vi "Main.vi"() -> ()   [LabVIEW 2020]
uses:
  SP200-DQMH/Libraries/SP200/EC-Lab Development Package/dll_Functions.llb/OCVParameters.ctl
  Shutter-DQMH/Libraries/Shutter/Shutter State.ctl
  <vilib>/Analysis/1siggen.llb/Ramp Pattern by Delta.vi
  SMC100-DQMH/Libraries/SMC100/SMC100.lvlib
  <vilib>/Analysis/NI_AALBase.lvlib
  Shutter-DQMH/Libraries/Shutter/Shutter.lvlib
  SP200-DQMH/Libraries/SP200/SP200.lvlib
panel:
  in  "Data Interval":u32=500
  out "Current values":T1
  in  "OCV Parameters":T2={"Rest_time_T"=1.0, "Record_every_dE"=0.01, "Record_every_dT"=0.01, "E_Range"=3, "em"=1, "ce"=0, "tb"=2e-05} {"tb" min=2e-05 max=1 format="%^_3e"; "ce" items=["Standard", "CE to ground"]; "E_Range" items=["±2.5V", "±5V", "±10V", "Auto"]; "Record_every_dT" min=0 format="%.2e"; "Record_every_dE" min=0 max=100 format="%.4f"; "Rest_time_T" min=0 format="%.2f"}
  in  "Channel":u8
  out "Path_t0":path=path "D:/LabVIEW/Delay-Shutter-Sync/Time_zero.txt"
  out "Relative Delay [ps]":dbl=1.0
  out "In Backstep":bool=TRUE
  out "Backstep pos.":dbl=-2.0
  in  "Backstep Delta [ps]":dbl=-5.0
  in  "Backstep":bool=TRUE
  out "Time Remaining [min]":dbl=125.0 format="%#.1f"
  out "Estimated time total [min]":dbl=144.0 format="%#.1f"
  out "c/2 mm/ps 2":dbl=0.15
  in  "Fine Steps [ps]":dbl=0.1 format="%#_6f"
  in  "Fine End [ps]":dbl=1.0
  in  "Fine Start [ps]":dbl=-0.4999999999999953
  in  "time steps [ps]":dbl=1.0 format="%#_6f"
  out "c/2 mm/ps":dbl=0.15
  in  "End delta t [ps]":dbl=30.0 format="%#_6f"
  in  "Start delta t [ps]":dbl=-5.0
  in  "Position Time zero":dbl=14.927
  in  "CLOSED Shutter Time (s)":dbl=50.0
  in  "Fine?":bool=TRUE
  in  "Fine Steps":dbl=0.0075 format="%#_6f"
  in  "Fine End":dbl=14.62325
  in  "Fine Start":dbl=14.39825
  out "Position":dbl=14.4432
  out "Shutter State":bool
  in  "Open Shutter Panel":bool
  in  "Open Delay Stage Panel":bool
  in  "SMC100 Serial Port":u8=3
  in  "Run":bool
  out "Seconds Running":i16
  in  "OPEN Shutter Time (s)":dbl=60.0
  out "Number of Steps":i32=72
  in  "Step Size":dbl=0.075 format="%#_6f"
  in  "End Position":dbl=17.47325
  in  "Start Position":dbl=14.17325
  in  "Exit":bool=TRUE
  # "Time"
  # "Space"
  # "Current"
  # "Control"
  # "Experiment"
  # "SP-200"
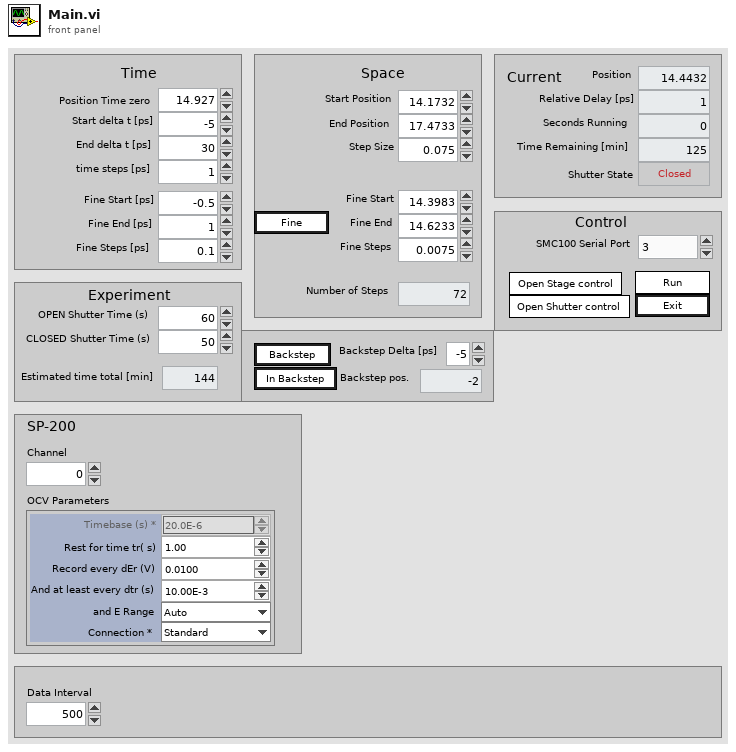
[diagram p1: front panel]
types:
  T1 = cluster{"State":i32, "MemFilled":i32, "TimeBase":sgl, " Ewe":sgl, " EweRangeMin":sgl, " EweRangeMax":sgl, "Ece":sgl, "EceRangeMin":sgl, "EceRangeMax":sgl, "Eoverflow":i32, "I":sgl, "IRange":i32, "Ioverflow":i32, "ElapsedTime":sgl, "Freq":sgl, "Rcomp":sgl, "Saturation":sgl, "OptErr":i32, "OptPos":i32}
  T2 = typedef "OCVParameters.ctl" = cluster{"Rest_time_T":sgl, "Record_every_dE":sgl, "Record_every_dT":sgl, "E_Range":u16, "em":u16, "ce":u16, "tb":sgl}
  T3 = enum32{"Invalid", "Standard", "Closed", "Hidden", "Minimized", "Maximized"}
  T4 = enum32{"invalid app kind", "Development System", "Run Time System", "Student Edition", "Embedded LabVIEW", "Evaluation", "Custom"}
  T5 = enum16{"open", "replace", "create", "open or create", "replace or create", "replace or create with confirmation"}
  T6 = typedef "Shutter State.ctl" = enum16{"None", "Open", "Closed"}
  T7 = enum8{"Enabled", "Disabled", "Disabled and Grayed Out"}
  T8 = cluster{"Core":cluster{"Current VI Reference":refnum<vi>, "Close Panel on Exit?":bool}, "Delay Positions":dbl[], "OPEN Shutter Time (s)":dbl, "Position Index":i32, "CLOSED Shutter Time (s)":dbl, "Shutter Close Time":u32, "Shutter Open Time":u32, "Save File Reference":refnum<file>}
  T9 = cluster{"Current VI Reference":refnum<vi>, "Close Panel on Exit?":bool}
  T10 = typedef "SMC100.lvlib/Get Abs Position (Reply Payload)--cluster.ctl" = cluster{"Absolute Position":dbl, "Get Abs Position_error":errorcluster}
  T11 = typedef "Shutter.lvlib/Get Shutter State (Reply Payload)--cluster.ctl" = cluster{"Shutter State":T6, "Get Shutter State_error":errorcluster}
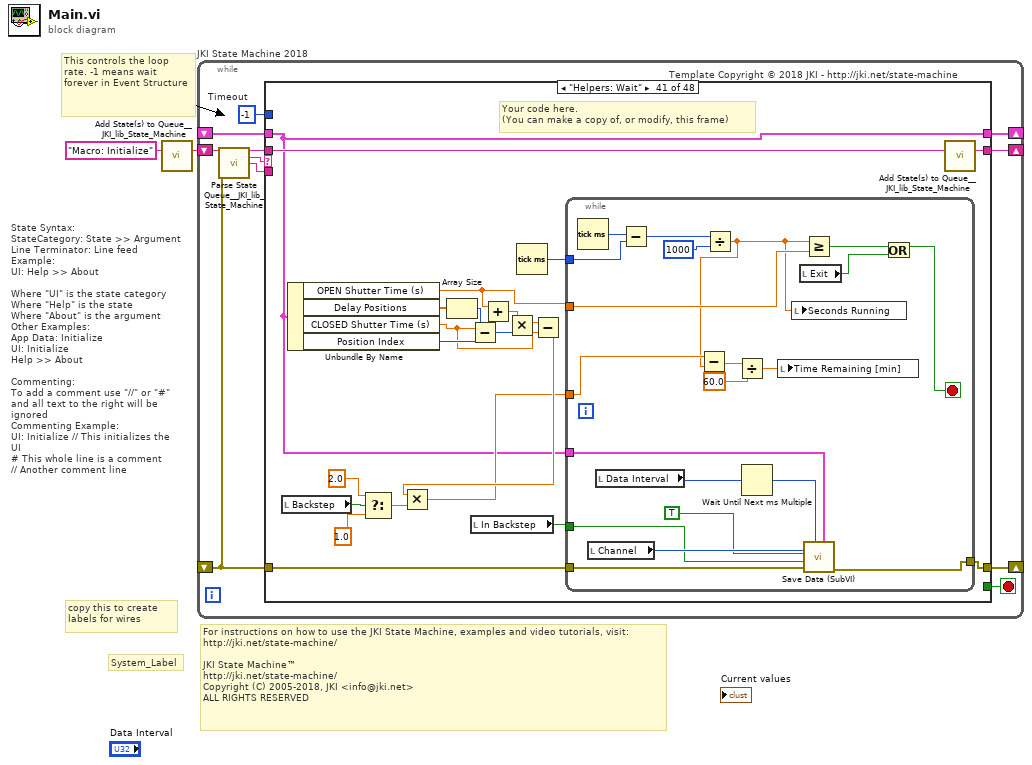
[diagram p0: block diagram]
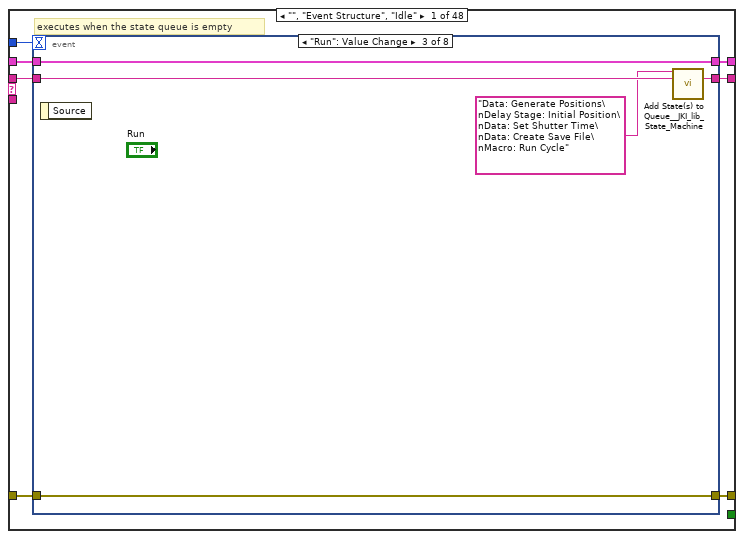
[diagram p2: hidden frame]
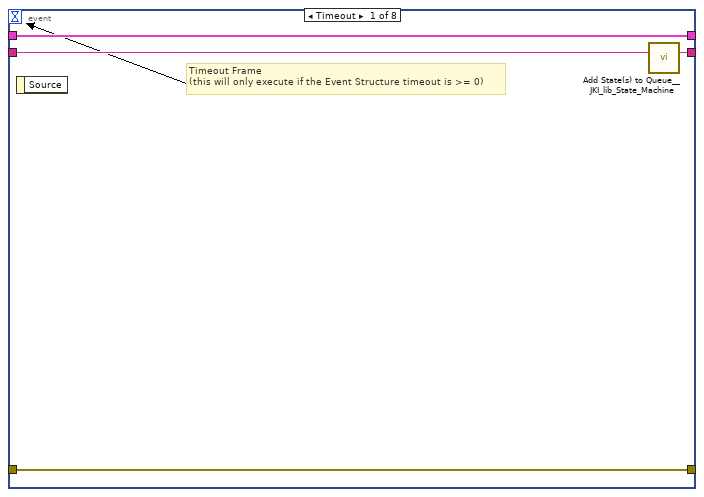
[diagram p3: hidden frame]
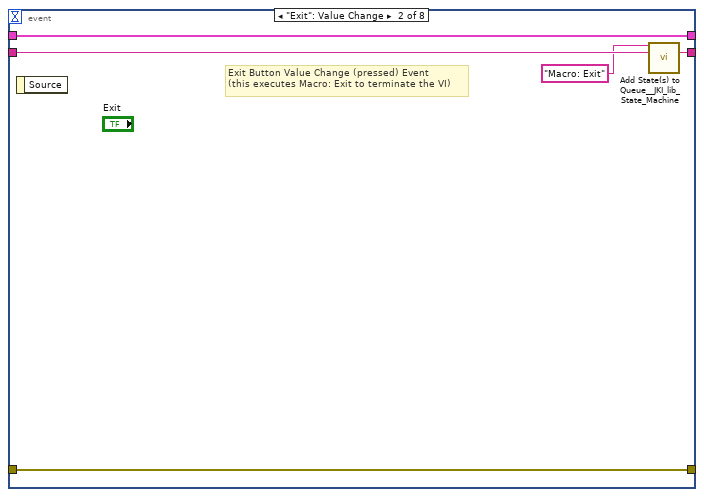
[diagram p4: hidden frame]
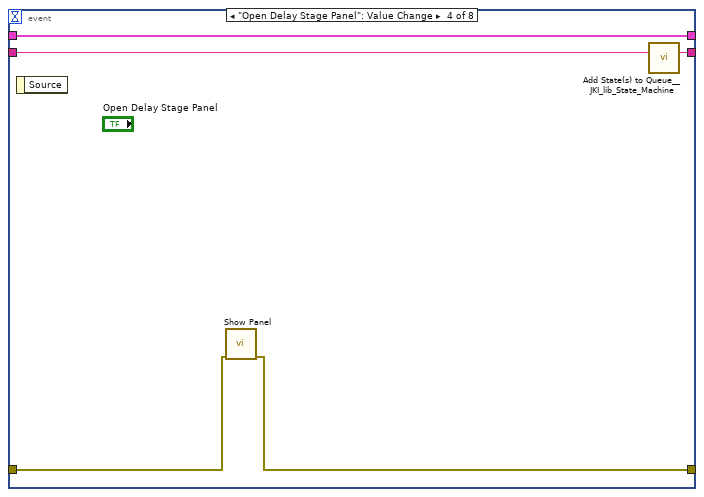
[diagram p5: hidden frame]
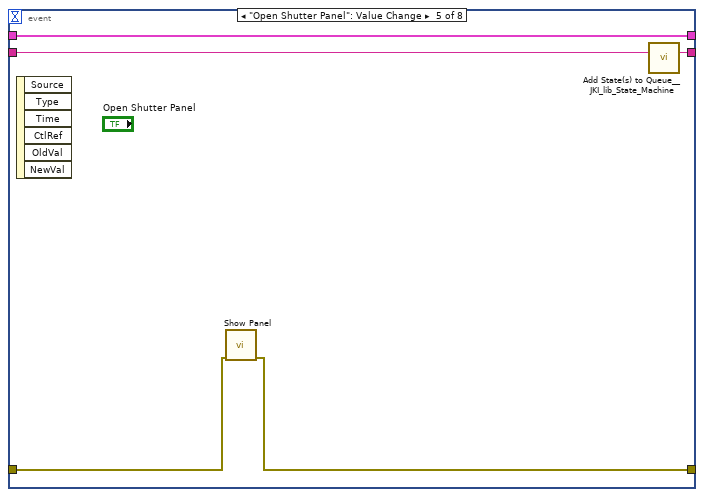
[diagram p6: hidden frame]
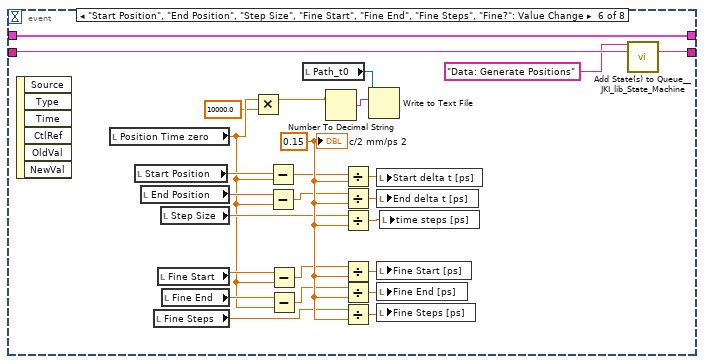
[diagram p7: hidden frame]
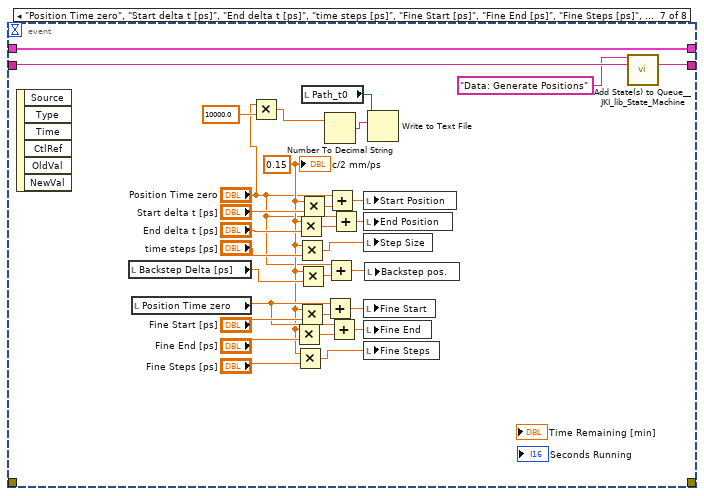
[diagram p8: hidden frame]
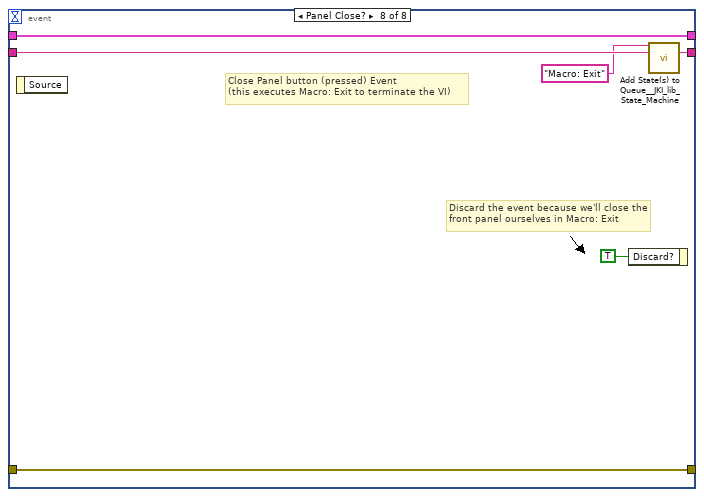
[diagram p9: hidden frame]
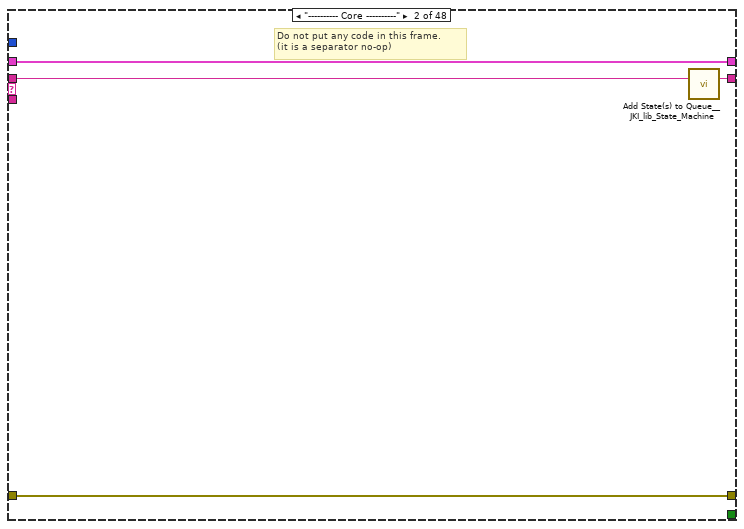
[diagram p10: hidden frame]
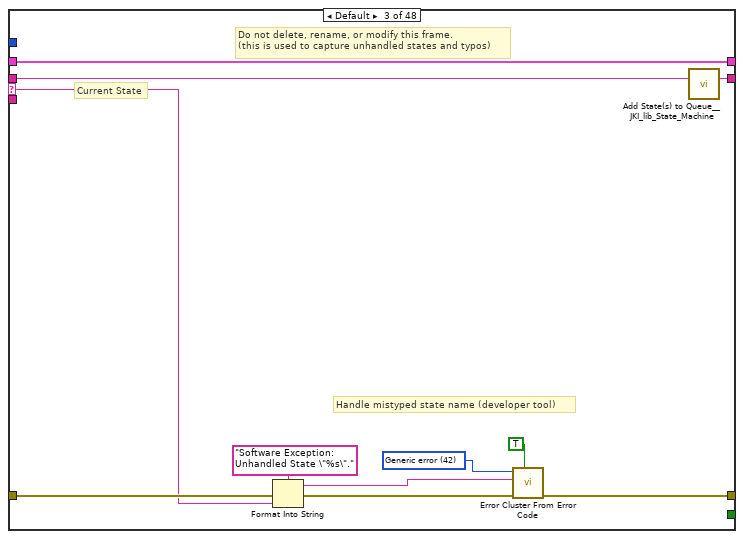
[diagram p11: hidden frame]
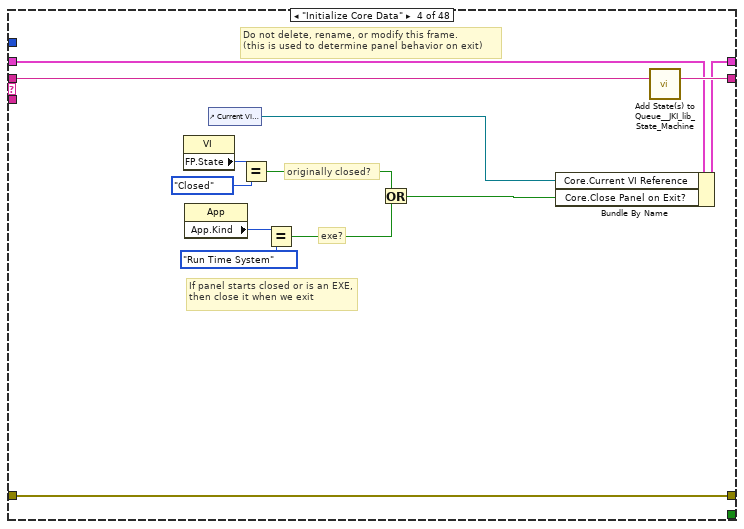
[diagram p12: hidden frame]
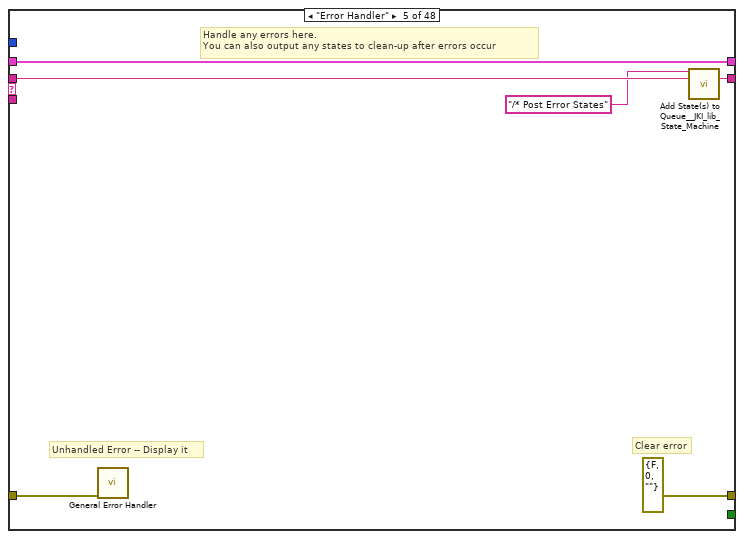
[diagram p13: hidden frame]
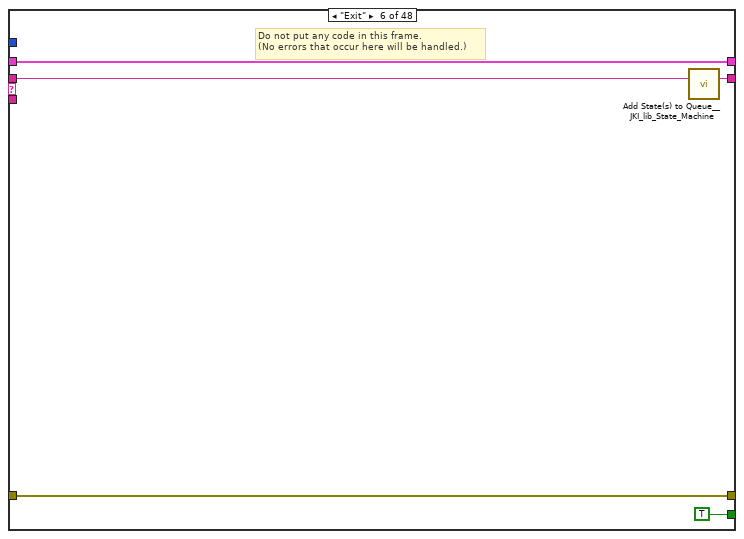
[diagram p14: hidden frame]
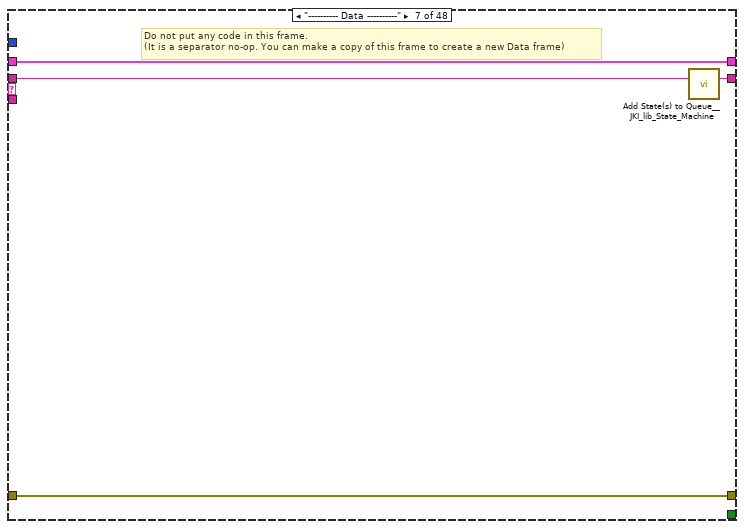
[diagram p15: hidden frame]
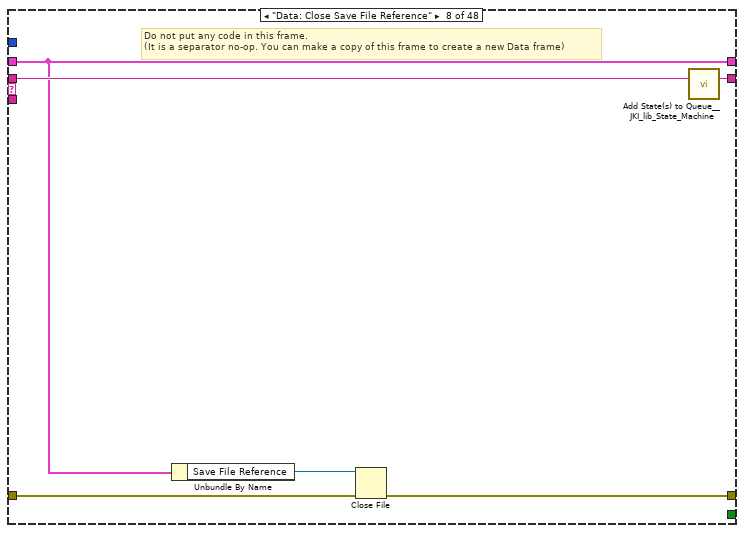
[diagram p16: hidden frame]
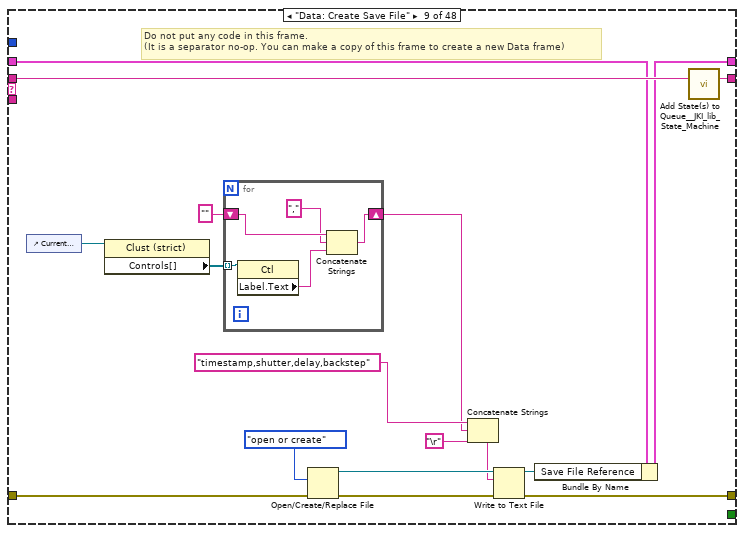
[diagram p17: hidden frame]
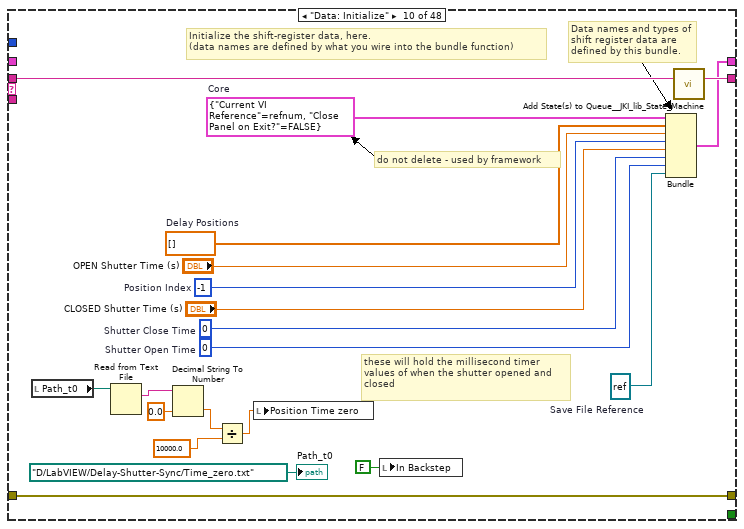
[diagram p18: hidden frame]
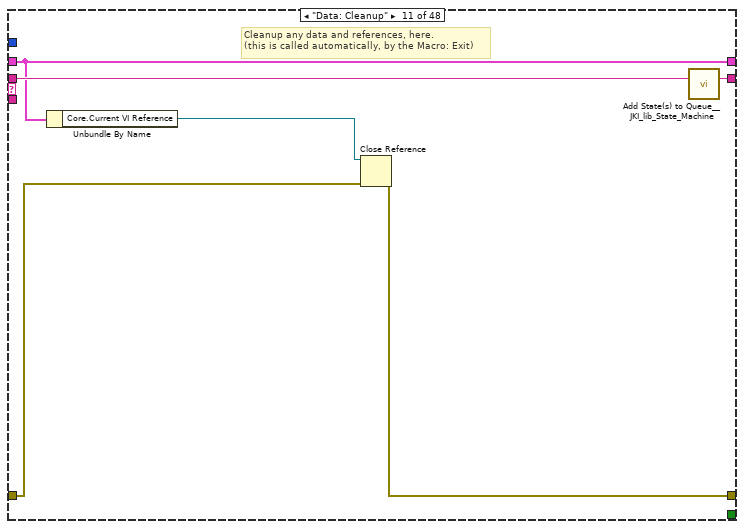
[diagram p19: hidden frame]
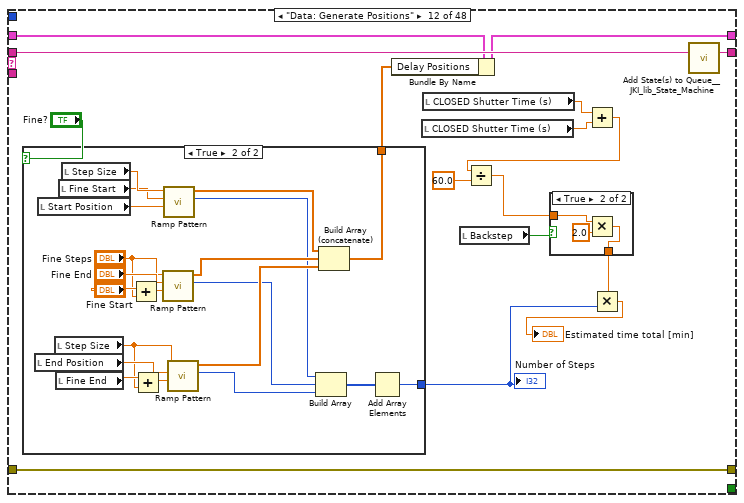
[diagram p20: hidden frame]
diagram:
  # "For instructions on how to use the JKI State Machine, examples and video tutorials, visit:\nhttp://jki.net/state-machine/\n\nJKI State Machine™\nhttp://jki.net/state-machine/\nCopyright (C) 2005-2018, JKI <info@jki.net>\nALL RIGHTS RESERVED"
  # "State Syntax:\nStateCategory: State >> Argument\nLine Terminator: Line feed\nExample:\nUI: Help >> About\n\nWhere \"UI\" is the state category\nWhere \"Help\" is the state\nWhere \"About\" is the argument\nOther Examples:\nApp Data: Initialize\nUI: Initialize\nHelp >> About\n\nCommenting:\nTo add a comment use \"//\" or \"#\" and all text to the right will be ignored\nCommenting Example:\nUI: Initialize // This initializes the UI\n# This whole line is a comment\n// Another comment line"
  # "copy this to create labels for wires"
  # "This controls the loop rate. -1 means wait forever in Event Structure"
  # "System_Label"
  n1 = call <vilib>:"Add State(s) to Queue__JKI_lib_State_Machine.vi"("State(s) in (\"\")"="Macro: Initialize") -> ("States Out"=w2:string)  [unwired: 14 in]
  n2 = while "JKI State Machine 2018" {
    shift-right: [w6] -> _
    shift-left: _ -> [w5]
    shift-right: [w9] -> _
    shift-left: _ -> [w3]
    shift-right: [w8] -> _
    shift-left: w2 -> [w10]
    stop <- w7 stop-if-true
    w4 = -1  # Timeout
    # "Template Copyright © 2018 JKI - http://jki.net/state-machine"
    n3 = call <vilib>:"Parse State Queue__JKI_lib_State_Machine.vi"("State Queue"=w10, "Error In (no error)"=w3) -> ("Remaining States"=w12:string, "Current State"=w13:string, "Arguments"=w11:string)  [unwired: 11 in]
    n4 = case shown="\"Helpers: Wait\"" w13 {
      selector: w13 -> [_ _ w111 _ _ _ _ _ _ _ _ _ _ _ _ _ _ _ _ _ _ _ _ _ _ _ _ _ _ _ _ _ _ _ _ _ _ _ _ _ _ _ _ _ _ _ _ _]
      tunnel: w12 -> [w20 w110 w115 w134 w140 w145 w149 w155 w172 w197 w203 w219 w256 w260 w264 w270 w281 w349 w355 w360 w365 w370 w375 w385 w390 w394 w400 w405 w411 w423 w435 w446 w450 w455 w460 w469 w478 w487 w491 w507 w537 w578 w603 w609 w618 w626 w631 w638]
      tunnel: w11 -> [_ _ _ _ _ _ _ _ _ _ _ _ _ _ _ w265 w275 _ _ _ _ _ _ _ _ _ _ _ _ _ _ _ _ _ _ _ _ _ _ _ _ _ _ _ _ _ _ _]
      tunnel: w5 -> [w18 w107 w113 w127 w137 w143 w146 w150 w169 _ w198 w216 w253 w257 w262 w268 w277 w348 w352 w357 w362 w367 w372 w382 w387 w391 w397 w402 w408 w419 w426 w443 w447 w452 w457 w466 w475 w485 w488 w504 w519 w561 w600 w607 w615 w623 w628 w635]
      tunnel: [w17 w108 w117 w131 errorcluster {"status"=FALSE, "code"=0, "source"=""} ("error out") w142 w147 w152 w166 w194 w199 w217 w254 w258 w261 w266 w278 w347 w353 w358 w363 w368 w373 w383 w388 w392 w396 w401 w407 w420 w432 w442 w448 w451 w456 w464 w474 w480 w489 w505 w520 w562 w601 w605 w612 w620 w627 w633] -> w9
      tunnel: w3 -> [w16 w108 w116 w131 w136 w142 w147 w153 w170 w194 w200 w217 w254 w258 w261 w267 w279 w347 w353 w358 w363 w368 w373 w383 w388 w392 w398 w403 w409 w421 w433 w444 w448 w453 w458 w467 w476 w481 w489 w505 w521 w563 w601 w606 w616 w624 w629 w636]
      tunnel: [w19 w109 w114 w133 w139 w144 w148 w154 w171 w196 w202 w218 w255 w259 w263 w269 w280 w350 w354 w359 w364 w369 w374 w384 w389 w393 w399 w404 w410 w422 w434 w445 w449 w454 w459 w468 w477 w486 w490 w506 w536 w577 w602 w608 w617 w625 w630 w637] -> w8
      tunnel: [_ _ _ _ _ TRUE _ _ _ _ _ _ _ _ _ _ _ _ _ _ _ _ _ _ _ _ _ _ _ _ _ _ _ _ _ _ _ _ _ _ _ _ _ _ _ _ _ _] -> w7
      tunnel: [w15 w107 w113 w132 w137 w143 w146 w150 w164 w195 w198 w215 w249 w257 w262 w268 w277 w348 w352 w357 w362 w367 w372 w382 w387 w391 w397 w402 w408 w417 w426 w443 w447 w452 w457 w462 w471 w485 w488 w501 w519 w561 w600 w607 w615 w623 w628 w635] -> w6
      tunnel: w4 -> [w14 _ _ _ _ _ _ _ _ _ _ _ _ _ _ _ _ _ _ _ _ _ _ _ _ _ _ _ _ _ _ _ _ _ _ _ _ _ _ _ _ _ _ _ _ _ _ _]
      frame "", "Event Structure", "Idle" {
        # "executes when the state queue is empty"
        n5 = event shown="[2] \"Run\": Value Change" {
          selector: _ -> [_ _ _ _ _ _ _ _]
          dyn-events: _ -> [_ _ _ _ _ _ _ _]
          timeout: w14 -> [_ _ _ _ _ _ _ _]
          tunnel: w20 -> [w24 w29 w34 w39 w44 w68 w98 w106]
          tunnel: [w23 w28 w33 w38 w43 w69 w99 w105] -> w19
          tunnel: w18 -> [w21 w26 w31 w37 w42 w70 w100 w103]
          tunnel: [w22 w27 w32 w36 w41 _ _ w104] -> w17
          tunnel: w16 -> [w22 w27 w32 w35 w40 _ _ w104]
          tunnel: [w21 w26 w31 w37 w42 w70 w100 w103] -> w15
          event Timeout {
            # "Timeout Frame\n(this will only execute if the Event Structure timeout is >= 0)"
            n6 = event-data() -> ()  [unwired: 1 in, 1 out]
            n7 = call <vilib>:"Add State(s) to Queue__JKI_lib_State_Machine.vi"("State(s) in (\"\")"=w24) -> ("States Out"=w23:string)  [unwired: 14 in]
          }
          event "Exit": Value Change {
            # "Exit Button Value Change (pressed) Event\n(this executes Macro: Exit to terminate the VI)"
            n8 = event-data() -> ()  [unwired: 1 in, 1 out]
            n9 = call <vilib>:"Add State(s) to Queue__JKI_lib_State_Machine.vi"("State(s) in Front (\"\")"="Macro: Exit", "State(s) in (\"\")"=w29) -> ("States Out"=w28:string)  [unwired: 13 in]
          }
          event "Run": Value Change {
            n10 = event-data() -> ()  [unwired: 1 in, 1 out]
            n11 = call <vilib>:"Add State(s) to Queue__JKI_lib_State_Machine.vi"("State(s) in Front (\"\")"="Data: Generate Positions\nDelay Stage: Initial Position\nData: Set Shutter Time\nData: Create Save File\nMacro: Run Cycle", "State(s) in (\"\")"=w34) -> ("States Out"=w33:string)  [unwired: 13 in]
          }
          event "Open Delay Stage Panel": Value Change {
            n12 = event-data() -> ()  [unwired: 1 in, 1 out]
            n13 = call "Show Panel.vi"("error in (no error)"=w35) -> ("error out"=w36:errorcluster)  [unwired: 10 in]
            n14 = call <vilib>:"Add State(s) to Queue__JKI_lib_State_Machine.vi"("State(s) in (\"\")"=w39) -> ("States Out"=w38:string)  [unwired: 14 in]
          }
          event "Open Shutter Panel": Value Change {
            n15 = event-data() -> ()  [unwired: 1 in, 6 out]
            n16 = call "Show Panel.vi"("error in (no error)"=w40) -> ("error out"=w41:errorcluster)  [unwired: 10 in]
            n17 = call <vilib>:"Add State(s) to Queue__JKI_lib_State_Machine.vi"("State(s) in (\"\")"=w44) -> ("States Out"=w43:string)  [unwired: 14 in]
          }
          event "Start Position", "End Position", "Step Size", "Fine Start", "Fine End", "Fine Steps", "Fine?": Value Change {
            w60 = 0.15 ("c mm/ps")
            n18 = event-data() -> ()  [unwired: 1 in, 6 out]
            n19 = local read "Position Time zero"() -> (w47:dbl)
            n20 = local read "Start Position"() -> (w59:dbl)
            n21 = local read "End Position"() -> (w58:dbl)
            n22 = local read "Fine Steps"() -> (w57:dbl)
            n23 = local read "Fine Start"() -> (w53:dbl)
            n24 = local read "Step Size"() -> (w56:dbl)
            n25 = local read "Fine End"() -> (w52:dbl)
            n26 = Multiply(x=w47, y=10000.0) -> (x*y=w46:dbl)
            n27 = Subtract(x=w59, y=w47) -> (x-y=w55:dbl)
            n28 = Subtract(x=w58, y=w47) -> (x-y=w54:dbl)
            n29 = Subtract(x=w53, y=w47) -> (x-y=w51:dbl)
            n30 = Subtract(x=w52, y=w47) -> (x-y=w50:dbl)
            n31 = local read "Path_t0"() -> (w48:path)
            n32 = Number To Decimal String(number=w46) -> (decimal integer string=w49:string)  [unwired: 1 in]
            n33 = Divide(x=w55, y=w60) -> (x/y=w66:dbl)
            n34 = Divide(x=w54, y=w60) -> (x/y=w64:dbl)
            n35 = Divide(x=w56, y=w60) -> (x/y=w65:dbl)
            n36 = Divide(x=w51, y=w60) -> (x/y=w61:dbl)
            n37 = Divide(x=w50, y=w60) -> (x/y=w62:dbl)
            n38 = Divide(x=w57, y=w60) -> (x/y=w63:dbl)
            n39 = Write to Text File(file (use dialog)=w48, text=w49) -> ()  [unwired: 2 in, 3 out]
            n40 = local write "Start delta t [ps]"(w66) -> ()
            n41 = local write "End delta t [ps]"(w64) -> ()
            n42 = local write "Fine Start [ps]"(w61) -> ()
            n43 = local write "Fine End [ps]"(w62) -> ()
            n44 = local write "Fine Steps [ps]"(w63) -> ()
            n45 = local write "time steps [ps]"(w65) -> ()
            n46 = call <vilib>:"Add State(s) to Queue__JKI_lib_State_Machine.vi"("State(s) in Front (\"\")"="Data: Generate Positions" ("State(s) in Front (\"\")"), "State(s) in (\"\")"=w68) -> ("States Out"=w69:string)  [unwired: 13 in]
            "c/2 mm/ps 2" <- w60
          }
          event "Position Time zero", "Start delta t [ps]", "End delta t [ps]", "time steps [ps]", "Fine Start [ps]", "Fine End [ps]", "Fine Steps [ps]", "CLOSED Shutter Time (s)", "OPEN Shutter Time (s)", "Backstep Delta [ps]": Value Change {
            w76 = 0.15 ("c mm/ps")
            n47 = event-data() -> ()  [unwired: 1 in, 6 out]
            n48 = local read "Backstep Delta [ps]"() -> (w77:dbl)
            n49 = local read "Position Time zero"() -> (w80:dbl)
            n50 = Multiply(x="Position Time zero", y=10000.0) -> (x*y=w71:dbl)
            n51 = Multiply(x=w76, y="Fine End [ps]") -> (x*y=w85:dbl)
            n52 = Multiply(x=w76, y="Fine Steps [ps]") -> (x*y=w88:dbl)
            n53 = Multiply(x=w76, y="End delta t [ps]") -> (x*y=w93:dbl)
            n54 = Multiply(x=w76, y="time steps [ps]") -> (x*y=w89:dbl)
            n55 = Multiply(x=w76, y="Fine Start [ps]") -> (x*y=w84:dbl)
            n56 = Multiply(x=w76, y=w77) -> (x*y=w78:dbl)
            n57 = Multiply(x=w76, y="Start delta t [ps]") -> (x*y=w95:dbl)
            n58 = local read "Path_t0"() -> (w74:path)
            n59 = Number To Decimal String(number=w71) -> (decimal integer string=w75:string)  [unwired: 1 in]
            n60 = Add(x=w80, y=w84) -> (x+y=w86:dbl)
            n61 = Add(x="Position Time zero", y=w78) -> (x+y=w79:dbl)
            n62 = Add(x="Position Time zero", y=w95) -> (x+y=w92:dbl)
            n63 = Add(x=w80, y=w85) -> (x+y=w87:dbl)
            n64 = Add(x="Position Time zero", y=w93) -> (x+y=w91:dbl)
            n65 = local write "Start Position"(w92) -> ()
            n66 = local write "End Position"(w91) -> ()
            n67 = local write "Step Size"(w89) -> ()
            n68 = local write "Fine Start"(w86) -> ()
            n69 = local write "Fine End"(w87) -> ()
            n70 = local write "Fine Steps"(w88) -> ()
            n71 = local write "Backstep pos."(w79) -> ()
            n72 = Write to Text File(file (use dialog)=w74, text=w75) -> ()  [unwired: 2 in, 3 out]
            n73 = call <vilib>:"Add State(s) to Queue__JKI_lib_State_Machine.vi"("State(s) in Front (\"\")"="Data: Generate Positions" ("State(s) in Front (\"\")"), "State(s) in (\"\")"=w98) -> ("States Out"=w99:string)  [unwired: 13 in]
            "c/2 mm/ps" <- w76
          }
          event Panel Close? {
            # "Discard the event because we'll close the front panel ourselves in Macro: Exit"
            # "Close Panel button (pressed) Event\n(this executes Macro: Exit to terminate the VI)"
            n74 = event-data() -> ()  [unwired: 1 in, 1 out]
            n75 = event-data("Discard?"=TRUE) -> ()  [unwired: 1 in, 1 out]
            n76 = call <vilib>:"Add State(s) to Queue__JKI_lib_State_Machine.vi"("State(s) in Front (\"\")"="Macro: Exit", "State(s) in (\"\")"=w106) -> ("States Out"=w105:string)  [unwired: 13 in]
          }
        }
      }
      frame "---------- Core ----------" {
        # "Do not put any code in this frame.\n(it is a separator no-op)"
        n77 = call <vilib>:"Add State(s) to Queue__JKI_lib_State_Machine.vi"("State(s) in (\"\")"=w110) -> ("States Out"=w109:string)  [unwired: 14 in]
      }
      frame Default {
        w120 = 42 items=["No error", "Argument error", "Memory is full", "Out of zone", "End of file", "File already open", "Generic file I/O error", "File not found", "File permission error", "Disk is full", "Duplicate path", "Too many files open", "System feature not enabled", "Resource file not found", "Cannot add resource", "Resource not found", "Image not found", "Image memory error", "Pen does not exist", "Config type invalid", "Config token not found", "Config parse error", "Config memory error", "Bad external code format", "Bad external code offset", "External code not present", "Null window", "Destroy window error", "Null menu", "Print aborted", "Bad print record", "Print driver error", "Windows error during printing", "Memory error during printing", "Print dialog error", "Generic print error", "Invalid device refnum", "Device not found", "Device parameter error", "Device unit error", "Cannot open device", "Device call aborted", "Generic error", "Cancelled by user", "Object ID too low", "Object ID too high", "Object not in heap", "Unknown heap", "Unknown object (invalid DefProc)", "Unknown object (DefProc not in table)", "Message out of range", "Invalid (null) method", "Unknown message", "Manager call not supported", "Bad address", "Network operation in progress", "Network operation timed out", "Connection is busy", "Network attribute not supported", "Network error", "Address in use", "System out of memory", "Connection aborted", "Connection refused", "Not connected", "Already connected", "Connection closed", "Initialization error (interapplication manager)", "Bad occurrence", "Wait on unbound occurrence handler", "Occurrence queue overflow", "Datalog type conflict", "Unused", "Unrecognized type (interapplication manager)", "Memory corrupt", "Failed to make temporary DLL", "Old CIN version", "Drag socket not found", "Failed to load drop-object", "Failed to register OLE object", "Failed to release OLE object", "Format specifier type mismatch", "Unknown format specifier", "Too few format specifiers", "Too many format specifiers", "Scan failed", "Newer CIN version", "Error converting to variant", "Runtime menu error", "Password tampered", "Variant attribute not found", "Incompatible variant data type", "Event data is not available", "Event Store is not present", "Occurrence is not found", "Event Queue is not created", "Event info is not available", "Refnum passed is NULL", "Error retrieving Class GUID", "Error retrieving CoClass GUID", "Error retrieving TypeLib GUID.", "Bad built application magic bytes.", "Specific driver is different from the specific driver associated with the Logical Name.", "There is no session opened to the class driver.", "Max Error", "MAX - Error with config objects", "MAX - Error loading configuration", "MAX - Group not supported"]
        # "Current State"
        # "Do not delete, rename, or modify this frame.\n(this is used to capture unhandled states and typos)"
        # "Handle mistyped state name (developer tool)"
        n78 = Format Into String(format string="Software Exception: Unhandled State \"%s\"." ("message"), error in=w116, w111) -> (resulting string=w119:string, error out=w118:errorcluster)  [unwired: 1 in]
        n79 = call <vilib>:"Error Cluster From Error Code.vi"("show call chain? (False)"=TRUE, "error in (no error)"=w118, "error message (\"\")"=w119, "error code (0)"=w120) -> ("error out"=w117:errorcluster)  [unwired: 5 in]
        n80 = call <vilib>:"Add State(s) to Queue__JKI_lib_State_Machine.vi"("State(s) in (\"\")"=w115) -> ("States Out"=w114:string)  [unwired: 14 in]
      }
      frame "Initialize Core Data" {
        # "Do not delete, rename, or modify this frame.\n(this is used to determine panel behavior on exit)"
        # "originally closed?"
        # "exe?"
        # "If panel starts closed or is an EXE, then close it when we exit"
        n81 = property class="VI"() -> ("FP.State"=w124:T3)  [unwired: 2 in, 2 out]
        n82 = property class="App"() -> ("App.Kind"=w130:T4)  [unwired: 2 in, 2 out]
        n83 = control-ref of="Current VI Reference"() -> (w125:refnum<vi>)
        n84 = Equal?(x=w124, y=T3."Closed" ("Front Panel Window:State")) -> (x = y?=w122:bool)
        n85 = Equal?(x=w130, y=T4."Run Time System" ("Application:Kind")) -> (x = y?=w128:bool)
        n86 = Or(x=w122, y=w128) -> (x .or. y?=w126:bool)
        n87 = Bundle By Name(cluster=w127, "Core.Current VI Reference"=w125, "Core.Close Panel on Exit?"=w126) -> (w132:T8)
        n88 = call <vilib>:"Add State(s) to Queue__JKI_lib_State_Machine.vi"("State(s) in (\"\")"=w134) -> ("States Out"=w133:string)  [unwired: 14 in]
      }
      frame "Error Handler" {
        # "Unhandled Error -- Display it"
        # "Handle any errors here.\nYou can also output any states to clean-up after errors occur"
        # "Clear error"
        n89 = call <vilib>:"General Error Handler.vi"("error in (no error)"=w136) -> ()  [unwired: 10 in, 5 out]
        n90 = call <vilib>:"Add State(s) to Queue__JKI_lib_State_Machine.vi"("State(s) in Front (\"\")"="/* Post Error States", "State(s) in (\"\")"=w140) -> ("States Out"=w139:string)  [unwired: 13 in]
      }
      frame "Exit" {
        # "Do not put any code in this frame.\n(No errors that occur here will be handled.)"
        n91 = call <vilib>:"Add State(s) to Queue__JKI_lib_State_Machine.vi"("State(s) in (\"\")"=w145) -> ("States Out"=w144:string)  [unwired: 14 in]
      }
      frame "---------- Data ----------" {
        # "Do not put any code in this frame.\n(It is a separator no-op. You can make a copy of this frame to create a new Data frame)"
        n92 = call <vilib>:"Add State(s) to Queue__JKI_lib_State_Machine.vi"("State(s) in (\"\")"=w149) -> ("States Out"=w148:string)  [unwired: 14 in]
      }
      frame "Data: Close Save File Reference" {
        # "Do not put any code in this frame.\n(It is a separator no-op. You can make a copy of this frame to create a new Data frame)"
        n93 = Unbundle By Name(w150) -> ("Save File Reference"=w151:refnum<file>)
        n94 = Close File(refnum=w151, error in=w153) -> (error out=w152:errorcluster)  [unwired: 1 out]
        n95 = call <vilib>:"Add State(s) to Queue__JKI_lib_State_Machine.vi"("State(s) in (\"\")"=w155) -> ("States Out"=w154:string)  [unwired: 14 in]
      }
      frame "Data: Create Save File" {
        # "Do not put any code in this frame.\n(It is a separator no-op. You can make a copy of this frame to create a new Data frame)"
        n96 = control-ref of="Current values"() -> (w162:refnum<vi>)
        n97 = property class="Clust (strict)"(reference=w162) -> ("Controls[]"=w161:refnum<vi>[])  [unwired: 1 in, 2 out]
        n98 = for {
          tunnel: w161 -> [w177] mode=indexing
          shift-right: [w176] -> w158
          shift-left: "" -> [w175]
          n99 = property class="Ctl"(reference=w177) -> ("Label.Text"=w173:string)  [unwired: 1 in, 2 out]
          n100 = Concatenate Strings(w175, "," ("string"), w173) -> (w176:string)
        }
        n101 = Open/Create/Replace File(error in=w170, operation (0:open)=T5."open or create") -> (refnum out=w165:refnum<file>, error out=w168:errorcluster)  [unwired: 4 in, 1 out]
        n102 = Concatenate Strings("timestamp,shutter,delay,backstep" ("text"), w158, "\r") -> (w156:string)
        n103 = Write to Text File(file (use dialog)=w165, text=w156, error in=w168) -> (refnum out=w163:refnum<file>, error out=w166:errorcluster)  [unwired: 1 in, 1 out]
        n104 = Bundle By Name(cluster=w169, "Save File Reference"=w163) -> (w164:T8)
        n105 = call <vilib>:"Add State(s) to Queue__JKI_lib_State_Machine.vi"("State(s) in (\"\")"=w172) -> ("States Out"=w171:string)  [unwired: 14 in]
      }
      frame "Data: Initialize" {
        w178 = refnum<file> refnum  # Save File Reference
        w179 = u32 0  # Shutter Open Time
        w180 = u32 0  # Shutter Close Time
        w191 = -1  # Position Index
        w192 = dbl[] []  # Delay Positions
        w193 = T9 {"Current VI Reference"=refnum, "Close Panel on Exit?"=FALSE}  # Core
        # "these will hold the millisecond timer\nvalues of when the shutter opened and\nclosed"
        # "do not delete - used by framework"
        # "Data names and types of shift register data are defined by this bundle."
        # "Initialize the shift-register data, here.\n(data names are defined by what you wire into the bundle function)"
        n106 = local read "Path_t0"() -> (w186:path)
        n107 = Read from Text File(file (use dialog)=w186) -> (text=w185:string)  [unwired: 3 in, 3 out]
        n108 = Decimal String To Number(string=w185, default (0L)=0.0 ("default (0 I32)")) -> (number=w183:dbl)  [unwired: 1 in, 1 out]
        n109 = Divide(x=w183, y=10000.0 ("x/y")) -> (x/y=w182:dbl)
        n110 = local write "Position Time zero"(w182) -> ()
        n111 = local write "In Backstep"(FALSE ("In Backstep")) -> ()
        n112 = Bundle("Core"=w193, "Delay Positions"=w192, "OPEN Shutter Time (s)"="OPEN Shutter Time (s)", "Position Index"=w191, "CLOSED Shutter Time (s)"="CLOSED Shutter Time (s)", "Shutter Close Time"=w180, "Shutter Open Time"=w179, "Save File Reference"=w178) -> (w195:T8)  [unwired: 1 in]
        n113 = call <vilib>:"Add State(s) to Queue__JKI_lib_State_Machine.vi"("State(s) in (\"\")"=w197) -> ("States Out"=w196:string)  [unwired: 14 in]
        "Path_t0" <- path "D:/LabVIEW/Delay-Shutter-Sync/Time_zero.txt" ("file (use dialog)")
      }
      frame "Data: Cleanup" {
        # "Cleanup any data and references, here.\n(this is called automatically, by the Macro: Exit)"
        n114 = Unbundle By Name(w198) -> ("Core.Current VI Reference"=w201:refnum<vi>)
        n115 = Close Reference(reference=w201, error in (no error)=w200) -> (error out=w199:errorcluster)
        n116 = call <vilib>:"Add State(s) to Queue__JKI_lib_State_Machine.vi"("State(s) in (\"\")"=w203) -> ("States Out"=w202:string)  [unwired: 14 in]
      }
      frame "Data: Generate Positions" {
        n117 = case shown="True" "Fine?" {
          tunnel: [w225 w230] -> w208
          tunnel: [w224 w229] -> w213
          frame False {
            n118 = local read "Start Position"() -> (w226:dbl)
            n119 = call-poly <vilib>:"Ramp Pattern.vi"("start"=w226, "end"="End Position", "delta"="Step Size") -> ("samples"=w225:i32, "Ramp Pattern"=w224:dbl[])  [unwired: 6 in, 1 out]
          }
          frame True {
            n120 = local read "End Position"() -> (w241:dbl)
            n121 = local read "Start Position"() -> (w246:dbl)
            n122 = local read "Step Size"() -> (w238:dbl)
            n123 = local read "Fine End"() -> (w240:dbl)
            n124 = local read "Fine Start"() -> (w244:dbl)
            n125 = local read "Step Size"() -> (w245:dbl)
            n126 = Add(x="Fine Start", y="Fine Steps") -> (x+y=w243:dbl)
            n127 = Add(x=w240, y=w238) -> (x+y=w239:dbl)
            n128 = call-poly <vilib>:"Ramp Pattern.vi"("start"=w243, "end"="Fine End", "delta"="Fine Steps") -> ("samples"=w233:i32, "Ramp Pattern"=w236:dbl[])  [unwired: 6 in, 1 out]
            n129 = call-poly <vilib>:"Ramp Pattern.vi"("start"=w246, "end"=w244, "delta"=w245) -> ("samples"=w232:i32, "Ramp Pattern"=w237:dbl[])  [unwired: 6 in, 1 out]
            n130 = call-poly <vilib>:"Ramp Pattern.vi"("start"=w239, "end"=w241, "delta"=w238) -> ("samples"=w234:i32, "Ramp Pattern"=w235:dbl[])  [unwired: 6 in, 1 out]
            n131 = Build Array(w232, w233, w234) -> (w231:i32[])
            n132 = Build Array (concatenate)(w237, w236, w235) -> (w229:dbl[])
            n133 = Add Array Elements(numeric array=w231) -> (sum=w230:i32)
          }
        }
        "Number of Steps" <- w208
        n134 = Bundle By Name(cluster=w216, "Delay Positions"=w213) -> (w215:T8)
        n135 = local read "CLOSED Shutter Time (s)"() -> (w211:dbl)
        n136 = local read "CLOSED Shutter Time (s)"() -> (w212:dbl)
        n137 = local read "Backstep"() -> (w204:bool)
        n138 = Add(x=w212, y=w211) -> (x+y=w209:dbl)
        n139 = Divide(x=w209, y=60.0) -> (x/y=w206:dbl)
        n140 = case shown="True" w204 {
          tunnel: w206 -> [w220 w222]
          tunnel: [w220 w221] -> w205
          frame False {
          }
          frame True {
            n141 = Multiply(x=w222, y=2.0) -> (x*y=w221:dbl)
          }
        }
        n142 = Multiply(x=w205, y=w208) -> (x*y=→"Estimated time total [min]":dbl)
        n143 = call <vilib>:"Add State(s) to Queue__JKI_lib_State_Machine.vi"("State(s) in (\"\")"=w219) -> ("States Out"=w218:string)  [unwired: 14 in]
      }
      frame "Data: Set Shutter Time" {
        # "Do not put any code in this frame.\n(It is a separator no-op. You can make a copy of this frame to create a new Data frame)"
        n144 = local read "OPEN Shutter Time (s)"() -> (w252:dbl)
        n145 = local read "CLOSED Shutter Time (s)"() -> (w251:dbl)
        n146 = Bundle By Name(cluster=w253, "OPEN Shutter Time (s)"=w252) -> (w250:T8)
        n147 = Bundle By Name(cluster=w250, "CLOSED Shutter Time (s)"=w251) -> (w249:T8)
        n148 = call <vilib>:"Add State(s) to Queue__JKI_lib_State_Machine.vi"("State(s) in (\"\")"=w256) -> ("States Out"=w255:string)  [unwired: 14 in]
      }
      frame "---------- UI ----------" {
        # "Do not put any code in this frame.\n(It is a separator no-op. You can make a copy of this frame to create a new UI frame)"
        n149 = call <vilib>:"Add State(s) to Queue__JKI_lib_State_Machine.vi"("State(s) in (\"\")"=w260) -> ("States Out"=w259:string)  [unwired: 14 in]
      }
      frame "UI: Initialize" {
        # "Initialize the User Interface, here.\n(this is called automatically, by the Macro: Init)"
        n150 = call <vilib>:"Add State(s) to Queue__JKI_lib_State_Machine.vi"("State(s) in (\"\")"=w264) -> ("States Out"=w263:string)  [unwired: 14 in]
      }
      frame "UI: Cursor Set" {
        # "Argument"
        # "Set and Unset Cursor Busy.\n(Usage: \"UI: Cursor Set >> Busy|Idle\")"
        n151 = case shown="\"Idle\", Default" w265 {
          tunnel: w267 -> [w272 w274]
          tunnel: [w271 w273] -> w266
          frame "Idle", Default {
            n152 = call <vilib>:"Unset Busy.vi"("error in (no error)"=w272) -> ("error out"=w271:errorcluster)  [unwired: 10 in]
          }
          frame "Busy" {
            n153 = call <vilib>:"Set Busy.vi"("error in (no error)"=w274) -> ("error out"=w273:errorcluster)  [unwired: 9 in, 1 out]
          }
        }
        n154 = call <vilib>:"Add State(s) to Queue__JKI_lib_State_Machine.vi"("State(s) in (\"\")"=w270) -> ("States Out"=w269:string)  [unwired: 14 in]
      }
      frame "UI: Front Panel State" {
        # "Argument"
        # "Set Front Panel Open or Closed\n(Usage: \"UI: Front Panel State >> Open|Close\")"
        n155 = Unbundle By Name(w277) -> ("Core.Current VI Reference"=w276:refnum<vi>)
        n156 = case shown="\"Minimize\", \"Minimized\"" w275 {
          tunnel: w279 -> [w287 w302 w313 w326 w339]
          tunnel: [w289 w303 w315 w328 w341] -> w278
          tunnel: w276 -> [w288 w300 w314 w327 w340]
          frame "Open", "Standard", Default {
            w282 = T3."Standard" ("State")
            n157 = property class="VI"(reference=w288, error in=w287) -> (reference out=w285:refnum<vi>, error out=w286:errorcluster, "FP.State"=w284:T3)
            n158 = Not Equal?(x=w284, y=w282) -> (x != y?=w283:bool)
            n159 = case shown="True" w283 {
              tunnel: [w293 w295] -> w289
              tunnel: w286 -> [w292 w295]
              tunnel: w285 -> [w291 _]
              tunnel: w282 -> [w290 _]
              frame True {
                n160 = invoke class="VI" method="FP.Open"(reference=w291, error in=w292, "Activate"=TRUE, "State"=w290) -> (error out=w293:errorcluster)  [unwired: 1 in, 4 out]
              }
              frame False {
              }
            }
          }
          frame "Close", "Closed" {
            n161 = property class="VI"(reference=w300, error in=w302) -> (reference out=w299:refnum<vi>, error out=w301:errorcluster, "FP.State"=w297:T3)
            n162 = Not Equal?(x=w297, y=T3."Closed" ("Front Panel Window:State")) -> (x != y?=w296:bool)
            n163 = case shown="True" w296 {
              tunnel: [w304 w307] -> w303
              tunnel: w301 -> [w304 w306]
              tunnel: w299 -> [_ w305]
              frame False {
              }
              frame True {
                n164 = invoke class="VI" method="FP.Close"(reference=w305, error in=w306) -> (error out=w307:errorcluster)  [unwired: 1 in, 2 out]
              }
            }
          }
          frame "Hidden", "Hide" {
            w308 = T3."Hidden" ("State")
            n165 = property class="VI"(reference=w314, error in=w313) -> (reference out=w311:refnum<vi>, error out=w312:errorcluster, "FP.State"=w310:T3)
            n166 = Not Equal?(x=w310, y=w308) -> (x != y?=w309:bool)
            n167 = case shown="True" w309 {
              tunnel: [w319 w320] -> w315
              tunnel: w312 -> [w318 w320]
              tunnel: w311 -> [w317 _]
              tunnel: w308 -> [w316 _]
              frame True {
                n168 = invoke class="VI" method="FP.Open"(reference=w317, error in=w318, "State"=w316) -> (error out=w319:errorcluster)  [unwired: 2 in, 4 out]
              }
              frame False {
              }
            }
          }
          frame "Minimize", "Minimized" {
            w321 = T3."Minimized" ("State")
            n169 = property class="VI"(reference=w327, error in=w326) -> (reference out=w324:refnum<vi>, error out=w325:errorcluster, "FP.State"=w323:T3)
            n170 = Not Equal?(x=w323, y=w321) -> (x != y?=w322:bool)
            n171 = case shown="True" w322 {
              tunnel: [w332 w333] -> w328
              tunnel: w325 -> [w331 w333]
              tunnel: w324 -> [w330 _]
              tunnel: w321 -> [w329 _]
              frame True {
                n172 = invoke class="VI" method="FP.Open"(reference=w330, error in=w331, "State"=w329) -> (error out=w332:errorcluster)  [unwired: 2 in, 4 out]
              }
              frame False {
              }
            }
          }
          frame "Maximize", "Maximized" {
            w334 = T3."Maximized" ("State")
            n173 = property class="VI"(reference=w340, error in=w339) -> (reference out=w337:refnum<vi>, error out=w338:errorcluster, "FP.State"=w336:T3)
            n174 = Not Equal?(x=w336, y=w334) -> (x != y?=w335:bool)
            n175 = case shown="True" w335 {
              tunnel: [w345 w346] -> w341
              tunnel: w338 -> [w344 w346]
              tunnel: w337 -> [w343 _]
              tunnel: w334 -> [w342 _]
              frame True {
                n176 = invoke class="VI" method="FP.Open"(reference=w343, error in=w344, "State"=w342) -> (error out=w345:errorcluster)  [unwired: 2 in, 4 out]
              }
              frame False {
              }
            }
          }
        }
        n177 = call <vilib>:"Add State(s) to Queue__JKI_lib_State_Machine.vi"("State(s) in (\"\")"=w281) -> ("States Out"=w280:string)  [unwired: 14 in]
      }
      frame "UI: Stop Exit" {
        n178 = local write "Exit"(FALSE ("Run")) -> ()
        n179 = call <vilib>:"Add State(s) to Queue__JKI_lib_State_Machine.vi"("State(s) in (\"\")"=w349) -> ("States Out"=w350:string)  [unwired: 14 in]
      }
      frame "---------- Macro ----------" {
        # "Do not put any code in this frame.\n(It is a separator no-op. You can make a copy of this frame to create a new Macro frame)"
        n180 = call <vilib>:"Add State(s) to Queue__JKI_lib_State_Machine.vi"("State(s) in (\"\")"=w355) -> ("States Out"=w354:string)  [unwired: 14 in]
      }
      frame "Macro: Run Cycle" {
        n181 = call <vilib>:"Add State(s) to Queue__JKI_lib_State_Machine.vi"("State(s) in Front (\"\")"="Shutter: Close\nShutter: Get Shutter State\nDelay Stage: Move Next\nDelay Stage: Get Position\nHelpers: Wait Closed\nShutter: Open\nShutter: Get Shutter State\nHelpers: Wait\nHelpers: At End?" ("State(s) in Front (\"\")"), "State(s) in (\"\")"=w360) -> ("States Out"=w359:string)  [unwired: 13 in]
      }
      frame "Macro: Backstep" {
        n182 = call <vilib>:"Add State(s) to Queue__JKI_lib_State_Machine.vi"("State(s) in Front (\"\")"="Shutter: Close\nShutter: Get Shutter State\nDelay Stage: Move Back\nDelay Stage: Get Position\nHelpers: Wait Closed\nShutter: Open\nShutter: Get Shutter State\nHelpers: Wait\nHelpers: At End?" ("State(s) in Front (\"\")"), "State(s) in (\"\")"=w365) -> ("States Out"=w364:string)  [unwired: 13 in]
      }
      frame "Macro: Initialize" {
        # "Initialization Macro\n(This is called once, when the VI starts)"
        n183 = call <vilib>:"Add State(s) to Queue__JKI_lib_State_Machine.vi"("State(s) in Front (\"\")"="Data: Initialize\nInitialize Core Data\nDelay Stage: Start Module\nShutter: Start Module\nSP 200: Start Module\nUI: Initialize\nUI: Front Panel State >> Open\nUI: Stop Exit", "State(s) in (\"\")"=w370) -> ("States Out"=w369:string)  [unwired: 13 in]
      }
      frame "Macro: Initial Device States" {
        n184 = call <vilib>:"Add State(s) to Queue__JKI_lib_State_Machine.vi"("State(s) in Front (\"\")"="Delay Stage: Initial Position\nSP 200: Set OCV Parameters\nSP 200: Start Channel" ("State(s) in Front (\"\")"), "State(s) in (\"\")"=w375) -> ("States Out"=w374:string)  [unwired: 13 in]
      }
      frame "Macro: Exit" {
        # "Exit Macro\n(This is called once, when the VI exits)"
        n185 = Unbundle By Name(w382) -> ("Core.Close Panel on Exit?"=w381:bool)
        n186 = Select(t="UI: Front Panel State >> Close", s=w381, f="") -> (s? t:f=w378:string)
        n187 = call <vilib>:"Add State(s) to Queue__JKI_lib_State_Machine.vi"("State(s) in (\"\")"=w378, "State(s) at Back (\"\")"="Delay Stage: Stop Module\nShutter: Stop Module\nSP 200: Stop Module\nData: Cleanup\nExit") -> ("States Out"=w376:string)  [unwired: 13 in]
        n188 = call <vilib>:"Add State(s) to Queue__JKI_lib_State_Machine.vi"("State(s) in Front (\"\")"=w376, "State(s) in (\"\")"=w385) -> ("States Out"=w384:string)  [unwired: 13 in]
      }
      frame "Macro: Device Cleanup" {
        # "Do not put any code in this frame.\n(It is a separator no-op. You can make a copy of this frame to create a new Macro frame)"
        n189 = call <vilib>:"Add State(s) to Queue__JKI_lib_State_Machine.vi"("State(s) in Front (\"\")"="Data: Close Save File Reference\nShutter: Close\nShutter: Get Shutter State\nDelay Stage: Get Position\nSP 200: Stop Channel\nUI: Stop Exit" ("State(s) in Front (\"\")"), "State(s) in (\"\")"=w390) -> ("States Out"=w389:string)  [unwired: 13 in]
      }
      frame "---------- Delay Stage ----------" {
        # "Template Separator\n(You can make a copy of, or modify, this frame)"
        n190 = call <vilib>:"Add State(s) to Queue__JKI_lib_State_Machine.vi"("State(s) in (\"\")"=w394) -> ("States Out"=w393:string)  [unwired: 14 in]
      }
      frame "Delay Stage: Start Module" {
        # "Template Separator\n(You can make a copy of, or modify, this frame)"
        n191 = call "Start Module.vi"("error in (no error)"=w398, "SerialPort"="SMC100 Serial Port") -> ("error out"=w396:errorcluster)  [unwired: 6 in, 3 out]
        n192 = call <vilib>:"Add State(s) to Queue__JKI_lib_State_Machine.vi"("State(s) in (\"\")"=w400) -> ("States Out"=w399:string)  [unwired: 14 in]
      }
      frame "Delay Stage: Stop Module" {
        # "Template Separator\n(You can make a copy of, or modify, this frame)"
        n193 = call "Stop Module.vi"("error in (no error)"=w403) -> ("error out"=w401:errorcluster)  [unwired: 10 in]
        n194 = call <vilib>:"Add State(s) to Queue__JKI_lib_State_Machine.vi"("State(s) in (\"\")"=w405) -> ("States Out"=w404:string)  [unwired: 14 in]
      }
      frame "Delay Stage: Initial Position" {
        # "Your code here.\n(You can make a copy of, or modify, this frame)"
        n195 = call "Set Abs Position.vi"("error in (no error)"=w409, "Abolute Position"="Start Position") -> ("error out"=w407:errorcluster)  [unwired: 9 in]
        n196 = call <vilib>:"Add State(s) to Queue__JKI_lib_State_Machine.vi"("State(s) in (\"\")"=w411) -> ("States Out"=w410:string)  [unwired: 14 in]
      }
      frame "Delay Stage: Move Next" {
        # "Your code here.\n(You can make a copy of, or modify, this frame)"
        n197 = Unbundle By Name(w419) -> ("Delay Positions"=w418:dbl[], "Position Index"=w416:i32)
        n198 = Increment(x=w416) -> (x+1=w415:i32)
        n199 = Bundle By Name(cluster=w419, "Position Index"=w415) -> (w417:T8)
        n200 = Index Array(array=w418, index=w415) -> (element=w414:dbl)
        n201 = local write "In Backstep"(FALSE ("In Backstep")) -> ()
        n202 = call "Set Abs Position.vi"("error in (no error)"=w421, "Abolute Position"=w414) -> ("error out"=w420:errorcluster)  [unwired: 9 in]
        n203 = Wait (ms)(milliseconds to wait=u32 10000) -> ()  [unwired: 1 out]
        n204 = call <vilib>:"Add State(s) to Queue__JKI_lib_State_Machine.vi"("State(s) in (\"\")"=w423) -> ("States Out"=w422:string)  [unwired: 14 in]
      }
      frame "Delay Stage: Move Back" {
        # "Your code here.\n(You can make a copy of, or modify, this frame)"
        n205 = local read "Position Time zero"() -> (w428:dbl)
        n206 = Multiply(x=0.15 ("c mm/ps"), y="Backstep Delta [ps]") -> (x*y=w430:dbl)
        n207 = Add(x=w428, y=w430) -> (x+y=w425:dbl)
        "Backstep pos." <- w425
        n208 = call "Set Abs Position.vi"("error in (no error)"=w433, "Abolute Position"=w425) -> ("error out"=w432:errorcluster)  [unwired: 9 in]
        n209 = Wait (ms)(milliseconds to wait=u32 10000) -> ()  [unwired: 1 out]
        n210 = call <vilib>:"Add State(s) to Queue__JKI_lib_State_Machine.vi"("State(s) in (\"\")"=w435) -> ("States Out"=w434:string)  [unwired: 14 in]
        "In Backstep" <- TRUE ("In Backstep")
      }
      frame "Delay Stage: Get Position" {
        # "Template Separator\n(You can make a copy of, or modify, this frame)"
        n211 = call "Get Abs Position.vi"("error in (no error)"=w444) -> ("error out"=w442:errorcluster, "Reply Payload"=w441:T10)  [unwired: 8 in, 1 out]
        n212 = local read "Position Time zero"() -> (w437:dbl)
        n213 = Unbundle By Name(w441) -> ("Absolute Position"=w436:dbl)
        "Position" <- w436
        n214 = local read "c/2 mm/ps"() -> (w439:dbl)
        n215 = Subtract(x=w436, y=w437) -> (x-y=w440:dbl)
        n216 = Divide(x=w440, y=w439) -> (x/y=→"Relative Delay [ps]":dbl)
        n217 = call <vilib>:"Add State(s) to Queue__JKI_lib_State_Machine.vi"("State(s) in (\"\")"=w446) -> ("States Out"=w445:string)  [unwired: 14 in]
      }
      frame "---------- Shutter ----------" {
        # "Your code here.\n(You can make a copy of, or modify, this frame)"
        n218 = call <vilib>:"Add State(s) to Queue__JKI_lib_State_Machine.vi"("State(s) in (\"\")"=w450) -> ("States Out"=w449:string)  [unwired: 14 in]
      }
      frame "Shutter: Start Module" {
        # "Your code here.\n(You can make a copy of, or modify, this frame)"
        n219 = call "Start Module.vi"("error in (no error)"=w453) -> ("error out"=w451:errorcluster)  [unwired: 7 in, 3 out]
        n220 = call <vilib>:"Add State(s) to Queue__JKI_lib_State_Machine.vi"("State(s) in (\"\")"=w455) -> ("States Out"=w454:string)  [unwired: 14 in]
      }
      frame "Shutter: Stop Module" {
        # "Your code here.\n(You can make a copy of, or modify, this frame)"
        n221 = call "Stop Module.vi"("error in (no error)"=w458) -> ("error out"=w456:errorcluster)  [unwired: 10 in]
        n222 = call <vilib>:"Add State(s) to Queue__JKI_lib_State_Machine.vi"("State(s) in (\"\")"=w460) -> ("States Out"=w459:string)  [unwired: 14 in]
      }
      frame "Shutter: Open" {
        # "Your code here.\n(You can make a copy of, or modify, this frame)"
        n223 = call "Set Shutter State.vi"("error in (no error)"=w467, "Shutter State"=Shutter_State."Open") -> ("error out"=w464:errorcluster)  [unwired: 7 in, 2 out]
        n224 = Wait (ms)(milliseconds to wait=u32 200) -> (millisecond timer value=w461:u32)
        n225 = Bundle By Name(cluster=w466, "Shutter Open Time"=w461) -> (w462:T8)
        n226 = call <vilib>:"Add State(s) to Queue__JKI_lib_State_Machine.vi"("State(s) in (\"\")"=w469) -> ("States Out"=w468:string)  [unwired: 14 in]
      }
      frame "Shutter: Close" {
        # "Your code here.\n(You can make a copy of, or modify, this frame)"
        n227 = call "Set Shutter State.vi"("error in (no error)"=w476, "Shutter State"=Shutter_State."Closed") -> ("error out"=w474:errorcluster)  [unwired: 7 in, 2 out]
        n228 = Wait (ms)(milliseconds to wait=u32 200) -> (millisecond timer value=w470:u32)
        n229 = Bundle By Name(cluster=w475, "Shutter Close Time"=w470) -> (w471:T8)
        n230 = call <vilib>:"Add State(s) to Queue__JKI_lib_State_Machine.vi"("State(s) in (\"\")"=w478) -> ("States Out"=w477:string)  [unwired: 14 in]
      }
      frame "Shutter: Get Shutter State" {
        # "Your code here.\n(You can make a copy of, or modify, this frame)"
        n231 = call "Get Shutter State.vi"("error in (no error)"=w481) -> ("error out"=w480:errorcluster, "Reply Payload"=w484:T11)  [unwired: 8 in, 1 out]
        n232 = Unbundle By Name(w484) -> ("Shutter State"=w483:T6)
        n233 = Equal?(x=Shutter_State."Open" ("Shutter State"), y=w483) -> (x = y?=→"Shutter State":bool)
        n234 = call <vilib>:"Add State(s) to Queue__JKI_lib_State_Machine.vi"("State(s) in (\"\")"=w487) -> ("States Out"=w486:string)  [unwired: 14 in]
      }
      frame "---------- Helpers ----------" {
        # "Your code here.\n(You can make a copy of, or modify, this frame)"
        n235 = call <vilib>:"Add State(s) to Queue__JKI_lib_State_Machine.vi"("State(s) in (\"\")"=w491) -> ("States Out"=w490:string)  [unwired: 14 in]
      }
      frame "Helpers: At End?" {
        # "Your code here.\n(You can make a copy of, or modify, this frame)"
        n236 = Unbundle By Name(w504) -> ("Position Index"=w498:i32, "Delay Positions"=w500:dbl[])
        n237 = case shown="True" "Backstep" {
          tunnel: ["Macro: Run Cycle" w509] -> w492
          frame False {
          }
          frame True {
            n238 = local read "In Backstep"() -> (w510:bool)
            n239 = Select(t="Macro: Run Cycle", s=w510, f="Macro: Backstep") -> (s? t:f=w509:string)
          }
        }
        n240 = Increment(x=w498) -> (x+1=w497:i32)
        n241 = Array Size(array=w500) -> (size(s)=w499:i32)
        n242 = Greater Or Equal?(x=w497, y=w499) -> (x >= y?=w496:bool)
        n243 = local read "Exit"() -> (w494:bool)
        n244 = Or(x=w494, y=w496) -> (x .or. y?=w495:bool)
        n245 = Select(t="Macro: Device Cleanup", s=w495, f=w492) -> (s? t:f=w502:string)
        n246 = case shown="True" w495 {
          tunnel: w504 -> [w513 w516]
          tunnel: [w513 w515] -> w501
          frame False {
          }
          frame True {
            n247 = Bundle By Name(cluster=w516, "Position Index"=0) -> (w515:T8)
          }
        }
        n248 = call <vilib>:"Add State(s) to Queue__JKI_lib_State_Machine.vi"("State(s) in Front (\"\")"=w502, "State(s) in (\"\")"=w507) -> ("States Out"=w506:string)  [unwired: 13 in]
      }
      frame "Helpers: Wait" {
        # "Your code here.\n(You can make a copy of, or modify, this frame)"
        n249 = local read "Backstep"() -> (w518:bool)
        n250 = Unbundle By Name(w519) -> ("OPEN Shutter Time (s)"=w531:dbl, "Delay Positions"=w534:dbl[], "CLOSED Shutter Time (s)"=w527:dbl, "Position Index"=w532:i32)
        n251 = Select(t=2.0 ("y"), s=w518, f=1.0) -> (s? t:f=w523:dbl)
        n252 = Array Size(array=w534) -> (size(s)=w533:i32)
        n253 = Subtract(x=w533, y=w532) -> (x-y=w529:i32)
        n254 = local read "In Backstep"() -> (w517:bool)
        n255 = Add(x=w531, y=w527) -> (x+y=w530:dbl)
        n256 = Multiply(x=w530, y=w529) -> (x*y=w528:dbl)
        n257 = Tick Count (ms)() -> (millisecond timer value=w535:u32)
        n258 = Subtract(x=w528, y=w527) -> (x-y=w526:dbl)
        n259 = Multiply(x=w526, y=w523) -> (x*y=w525:dbl)
        n260 = while {
          tunnel: w535 -> [w557]
          tunnel: w531 -> [w555]
          tunnel: w525 -> [w550]
          tunnel: w521 -> [w545]
          tunnel: [w543] -> w520
          tunnel: w519 -> [w540]
          tunnel: w517 -> [w539]
          stop <- w552 stop-if-true
          n261 = Tick Count (ms)() -> (millisecond timer value=w558:u32)
          n262 = local read "Channel"() -> (w544:u8)
          n263 = local read "Data Interval"() -> (w538:u32)
          n264 = Subtract(x=w558, y=w557) -> (x-y=w556:u32)
          n265 = Divide(x=w556, y=u32 1000) -> (x/y=w546:dbl)
          n266 = Subtract(x=w550, y=w546) -> (x-y=w549:dbl)
          n267 = Divide(x=w549, y=60.0) -> (x/y=w547:dbl)
          n268 = Wait Until Next ms Multiple(millisecond multiple=w538) -> (millisecond timer value=w542:u32)
          n269 = local write "Time Remaining [min]"(w547) -> ()
          n270 = local write "Seconds Running"(w546) -> ()
          n271 = local read "Exit"() -> (w551:bool)
          n272 = Greater Or Equal?(x=w546, y=w555) -> (x >= y?=w553:bool)
          n273 = call "Save Data (SubVI).vi"("Data"=w540, "Channel"=w544, "timestamp"=w542, "error in (no error)"=w545, "Backstep"=w539, "Shutter"=TRUE) -> ("error out"=w543:errorcluster)  [unwired: 5 in]
          n274 = Or(x=w553, y=w551) -> (x .or. y?=w552:bool)
        }
        n275 = call <vilib>:"Add State(s) to Queue__JKI_lib_State_Machine.vi"("State(s) in (\"\")"=w537) -> ("States Out"=w536:string)  [unwired: 14 in]
      }
      frame "Helpers: Wait Closed" {
        # "Your code here.\n(You can make a copy of, or modify, this frame)"
        n276 = Unbundle By Name(w561) -> ("OPEN Shutter Time (s)"=w570:dbl, "Delay Positions"=w575:dbl[], "CLOSED Shutter Time (s)"=w569:dbl, "Position Index"=w573:i32)
        n277 = local read "In Backstep"() -> (w559:bool)
        n278 = local read "Backstep"() -> (w560:bool)
        n279 = Select(t=2.0 ("y"), s=w560, f=1.0) -> (s? t:f=w568:dbl)
        n280 = Array Size(array=w575) -> (size(s)=w574:i32)
        n281 = Subtract(x=w574, y=w573) -> (x-y=w571:i32)
        n282 = Add(x=w570, y=w569) -> (x+y=w572:dbl)
        n283 = Tick Count (ms)() -> (millisecond timer value=w576:u32)
        n284 = Multiply(x=w572, y=w571) -> (x*y=w565:dbl)
        n285 = Multiply(x=w565, y=w568) -> (x*y=w564:dbl)
        n286 = while {
          tunnel: w576 -> [w598]
          tunnel: w569 -> [w596]
          tunnel: w564 -> [w591]
          tunnel: w563 -> [w586]
          tunnel: [w585] -> w562
          tunnel: w561 -> [w584]
          tunnel: w559 -> [w582]
          stop <- w593 stop-if-true
          n287 = Tick Count (ms)() -> (millisecond timer value=w599:u32)
          n288 = local read "Channel"() -> (w580:u8)
          n289 = local read "Data Interval"() -> (w579:u32)
          n290 = Subtract(x=w599, y=w598) -> (x-y=w597:u32)
          n291 = Divide(x=w597, y=u32 1000) -> (x/y=w587:dbl)
          n292 = Subtract(x=w591, y=w587) -> (x-y=w590:dbl)
          n293 = Wait Until Next ms Multiple(millisecond multiple=w579) -> (millisecond timer value=w581:u32)
          n294 = Divide(x=w590, y=60.0) -> (x/y=w588:dbl)
          n295 = local write "Time Remaining [min]"(w588) -> ()
          n296 = local write "Seconds Running"(w587) -> ()
          n297 = call "Save Data (SubVI).vi"("Data"=w584, "Channel"=w580, "timestamp"=w581, "error in (no error)"=w586, "Backstep"=w582, "Shutter"=FALSE) -> ("error out"=w585:errorcluster)  [unwired: 5 in]
          n298 = local read "Exit"() -> (w592:bool)
          n299 = Greater Or Equal?(x=w587, y=w596) -> (x >= y?=w594:bool)
          n300 = Or(x=w594, y=w592) -> (x .or. y?=w593:bool)
        }
        n301 = call <vilib>:"Add State(s) to Queue__JKI_lib_State_Machine.vi"("State(s) in (\"\")"=w578) -> ("States Out"=w577:string)  [unwired: 14 in]
      }
      frame "---------- SP 200 ----------" {
        # "Your code here.\n(You can make a copy of, or modify, this frame)"
        n302 = call <vilib>:"Add State(s) to Queue__JKI_lib_State_Machine.vi"("State(s) in (\"\")"=w603) -> ("States Out"=w602:string)  [unwired: 14 in]
      }
      frame "SP 200: Set OCV Parameters" {
        # "Your code here.\n(You can make a copy of, or modify, this frame)"
        n303 = call "Set OCV Parameters.vi"("error in (no error)"=w606, "OCV Parameters"="OCV Parameters") -> ("error out"=w605:errorcluster)  [unwired: 7 in, 2 out]
        n304 = call <vilib>:"Add State(s) to Queue__JKI_lib_State_Machine.vi"("State(s) in (\"\")"=w609) -> ("States Out"=w608:string)  [unwired: 14 in]
      }
      frame "SP 200: Stop Channel" {
        # "Your code here.\n(You can make a copy of, or modify, this frame)"
        n305 = local read "Channel"() -> (w614:u8)
        n306 = control-ref of="Channel"() -> (w611:refnum<vi>)
        n307 = call "Stop Channel.vi"("error in (no error)"=w616, "Channel"=w614) -> ("error out"=w613:errorcluster)  [unwired: 9 in]
        n308 = property on="Property Node" class="DigNum (strict)"(reference=w611, error in=w613, "DisabledEnum"=T7."Enabled" ("Disabled")) -> (error out=w612:errorcluster)  [unwired: 1 out]
        n309 = call <vilib>:"Add State(s) to Queue__JKI_lib_State_Machine.vi"("State(s) in (\"\")"=w618) -> ("States Out"=w617:string)  [unwired: 14 in]
      }
      frame "SP 200: Start Channel" {
        # "Disable the channel picker\nto avoid that the channel is changed\nduring the measurement and another\nchannel is stopped that was not started.\nIt will be enabled again when the channel\nis stopped."
        # "Your code here.\n(You can make a copy of, or modify, this frame)"
        n310 = call "Start Channel.vi"("error in (no error)"=w624, "Channel"="Channel") -> ("error out"=w621:errorcluster)  [unwired: 7 in, 2 out]
        n311 = property on="Channel" class="DigNum (strict)"(error in=w621, "DisabledEnum"=T7."Disabled and Grayed Out" ("Disabled")) -> (error out=w620:errorcluster)  [unwired: 1 in, 1 out]
        n312 = call <vilib>:"Add State(s) to Queue__JKI_lib_State_Machine.vi"("State(s) in (\"\")"=w626) -> ("States Out"=w625:string)  [unwired: 14 in]
      }
      frame "SP 200: Stop Module" {
        # "Your code here.\n(You can make a copy of, or modify, this frame)"
        n313 = call "Stop Module.vi"("error in (no error)"=w629) -> ("error out"=w627:errorcluster)  [unwired: 10 in]
        n314 = call <vilib>:"Add State(s) to Queue__JKI_lib_State_Machine.vi"("State(s) in (\"\")"=w631) -> ("States Out"=w630:string)  [unwired: 14 in]
      }
      frame "SP 200: Start Module" {
        # "Your code here.\n(You can make a copy of, or modify, this frame)"
        n315 = Two Button Dialog(message="Due to a bug in the Biologic EC-Lab Development\nPackage you have to manually start the SP-200 DQMH\nmodule. After the module started press 'ok'. If you\npress 'cancel' the module will not be loaded.") -> (T button?=w632:bool)  [unwired: 2 in]
        n316 = case shown="False" w632 {
          tunnel: w636 -> [w639 w641]
          tunnel: [w639 w640] -> w633
          frame False {
          }
          frame True {
            n317 = call "Start Module.vi"("error in (no error)"=w641) -> ("error out"=w640:errorcluster)  [unwired: 7 in, 3 out]
          }
        }
        n318 = call <vilib>:"Add State(s) to Queue__JKI_lib_State_Machine.vi"("State(s) in (\"\")"=w638) -> ("States Out"=w637:string)  [unwired: 14 in]
      }
    }
  }
